vi "_ROSDefinition.vi"() -> ()   [LabVIEW 2016]
doc: "Global ROS properties"
panel:
  out "MyIP":string
  out "Debug":string
  out "WriteQ":refnum<queue>[](array[refnum])
  out "Canceled":bool
  out "FIFOQ":refnum<queue>[](array[refnum])
  out "CmdQ":refnum<queue>[](array[refnum])
  in  "Service Prov Wait":i32=5000
  out "Topic Port":u16[](array[numeric])
  out "Topic History":string[](array[string])
  out "Master History":string[](array[string])
  in  "Watchdog":i32=5000
  out "Webpage Port":u16=6263
  out "Am Master?":bool
  in  "Queue Size":i32=10
  in  "TCP wait":i32=1000
  out "Servers":u16[](array[numeric])
  out "Robot There?":bool
  out "ROS Master":string="192.168.1.110:11311"
  # "Currently disabled"
  # "First port is the log server"
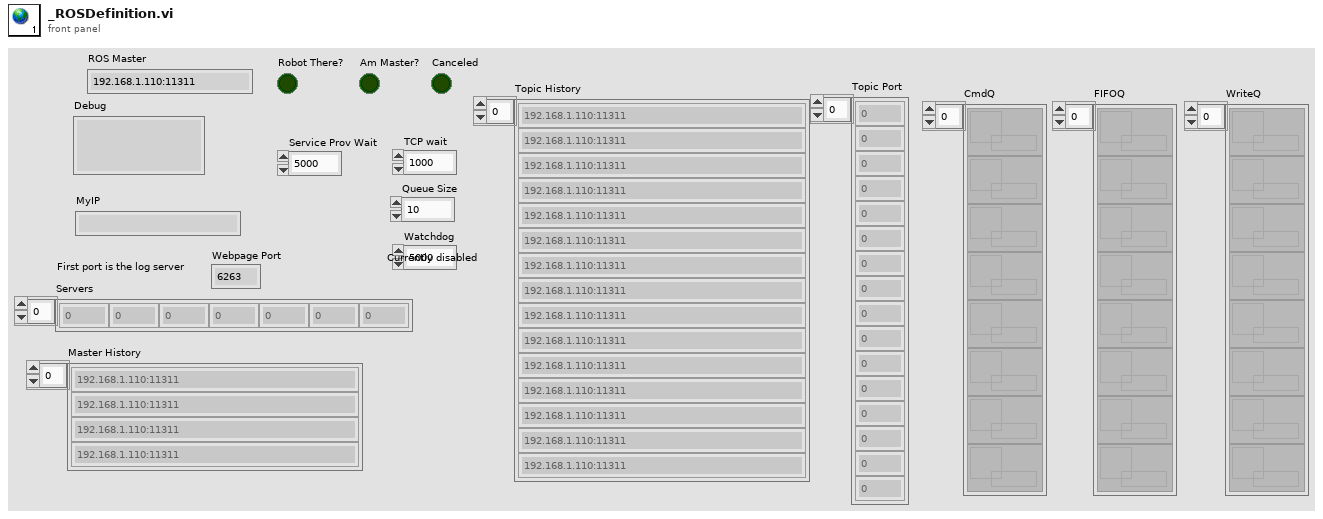
[diagram p1: front panel]
diagram:
